vi "csvtest.vi"(11 "path name":string) -> (2 "right path":dbl[][](array[numeric]), 3 "left path":dbl[][](array[numeric]))   [LabVIEW 2020]
uses:
  <vilib>/Utility/file.llb/Read Delimited Spreadsheet (DBL).vi
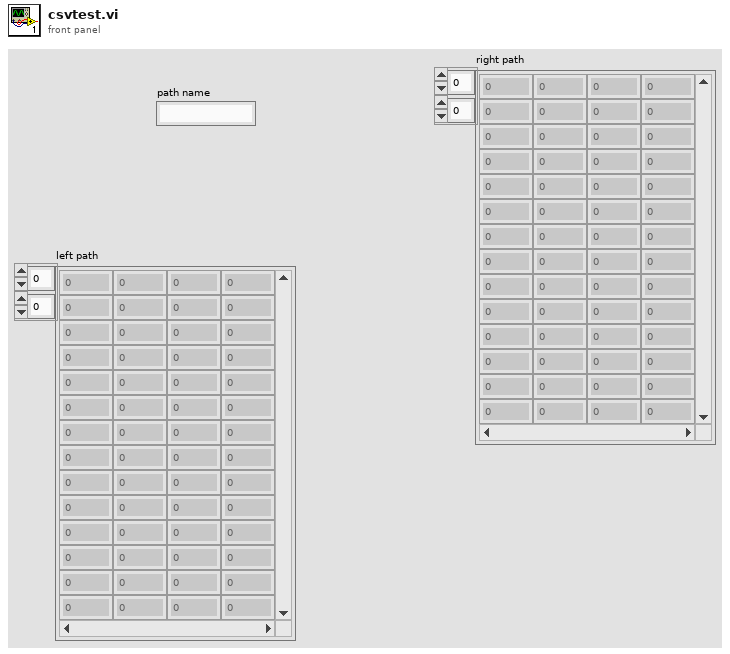
[diagram p1: front panel]
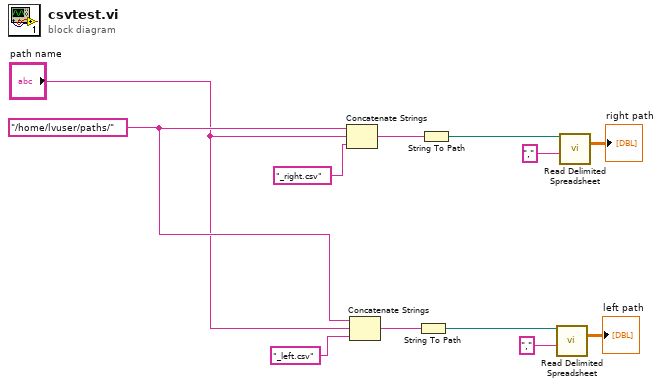
[diagram p0: block diagram]
diagram:
  w3 = "/home/lvuser/paths/" ("string")
  n1 = Concatenate Strings(w3, "path name", "_right.csv" ("string")) -> (w8:string)
  n2 = Concatenate Strings(w3, "path name", "_left.csv" ("string")) -> (w4:string)
  n3 = String To Path(string=w4) -> (path=w5:path)
  n4 = String To Path(string=w8) -> (path=w10:path)
  n5 = call-poly <vilib>:"Read Delimited Spreadsheet.vi"("file path (dialog if empty)"=w5, "delimiter (\\t)"="," ("delimiter (\\t)")) -> ("all rows"=→"left path":dbl[][])  [unwired: 8 in, 5 out]
  n6 = call-poly <vilib>:"Read Delimited Spreadsheet.vi"("file path (dialog if empty)"=w10, "delimiter (\\t)"="," ("delimiter (\\t)")) -> ("all rows"=→"right path":dbl[][])  [unwired: 8 in, 5 out]
